vi "saveData.vi"(1 "display write dialog?":bool, 2 "append to file?":bool, 3 "Block Timing":T1) -> (0 "error out":errorcluster)   [LabVIEW 2013]
uses:
  Controls/blockTiming.ctl
  Globals/measurementGlobal.vi
panel:
  out "File Status":string="File not appended"
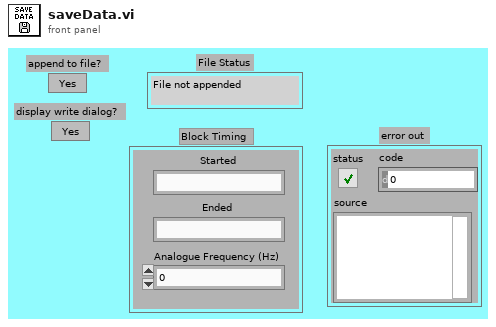
[diagram p1: front panel]
types:
  T1 = typedef "blockTiming.ctl" = cluster{"Started":string, "Ended":string, "Analogue Frequency (Hz)":dbl}
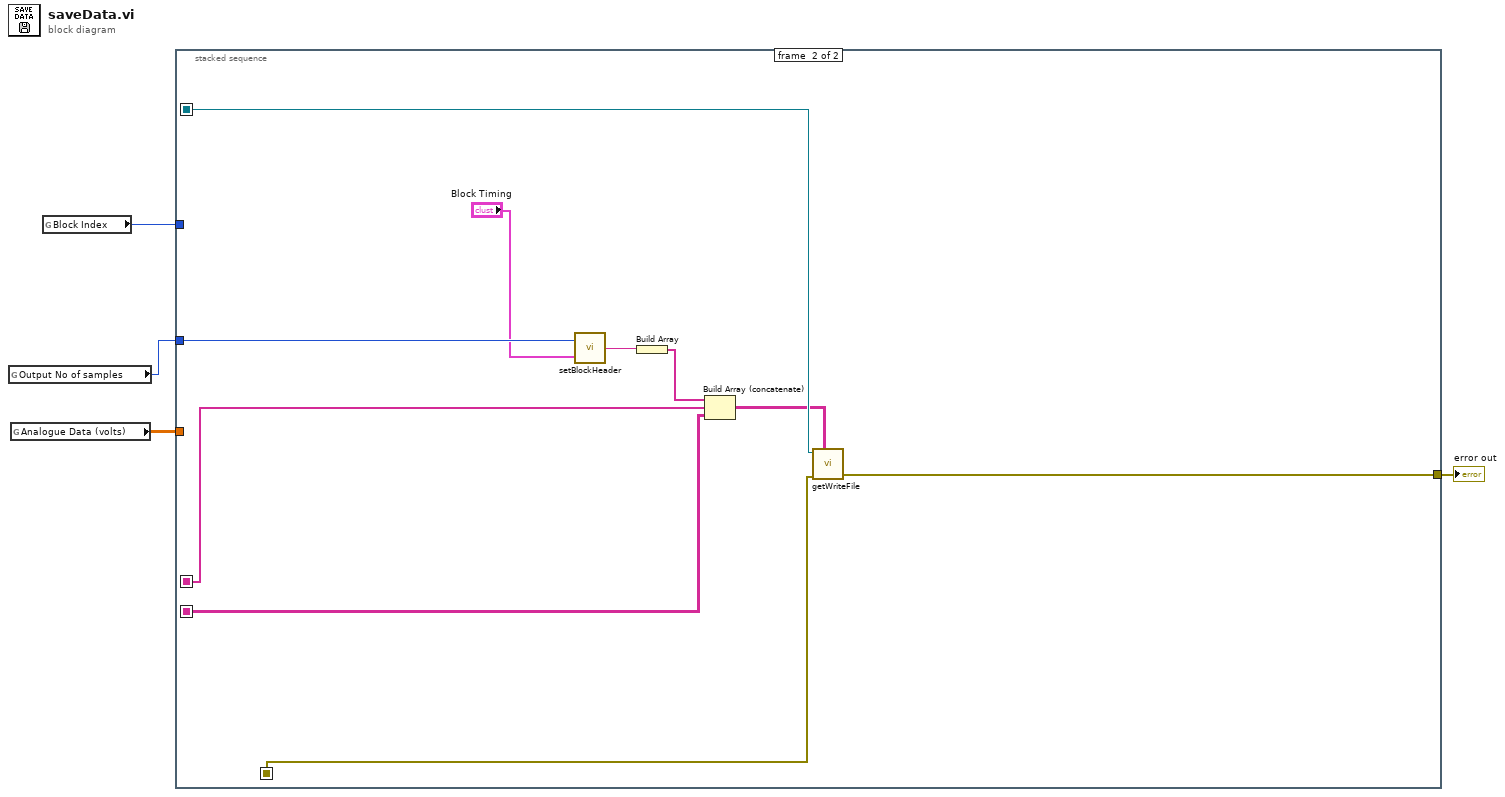
[diagram p0: block diagram]
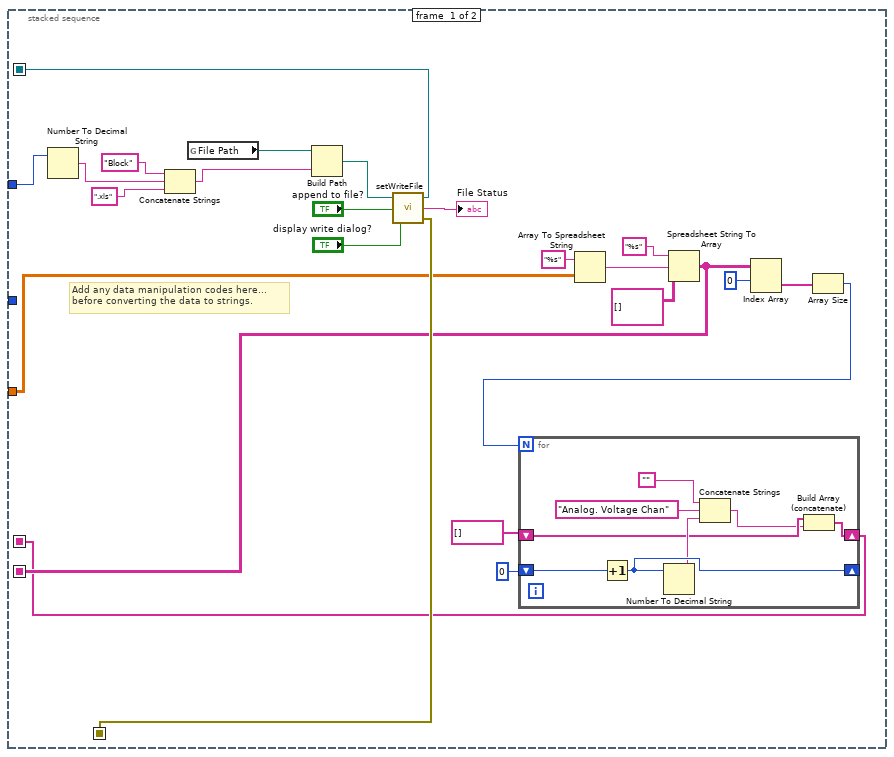
[diagram p2: hidden frame]
diagram:
  n1 = global read "measurementGlobal.vi" "Output No of samples"() -> (w3:i32)
  n2 = global read "measurementGlobal.vi" "Analogue Data (volts)"() -> (w4:dbl[][])
  n3 = global read "measurementGlobal.vi" "Block Index"() -> (w1:i32)
  n4 = stacked-sequence {
    seq-local: [w24 _] -> [_ w40]
    seq-local: [w23 _] -> [_ w39]
    seq-local: [w11 _] -> [_ w43]
    seq-local: [w10 _] -> [_ w44]
    tunnel: w4 -> [w19 _]
    tunnel: w3 -> [_ w46]
    tunnel: [_ w37] -> w2
    tunnel: w1 -> [w9 _]
    frame #0 {
      # "Add any data manipulation codes here... \nbefore converting the data to strings."
      n5 = Number To Decimal String(number=w9) -> (decimal integer string=w7:string)  [unwired: 1 in]
      n6 = Concatenate Strings("Block", w7, ".xls") -> (w5:string)
      n7 = global read "measurementGlobal.vi" "File Path"() -> (w28:path)
      n8 = Build Path(base path=w28, name or relative path=w5) -> (appended path=w27:path)
      n9 = call "setWriteFile.vi"("display write dialog?"="display write dialog?", "append to file?"="append to file?", "file path"=w27) -> ("error out"=w23:errorcluster, "Status"=→"File Status":string, "File Refnum"=w24:refnum<file>)
      n10 = Array To Spreadsheet String(array=w19, 3:"%s" ("format string")) -> (spreadsheet string=w15:string)  [unwired: 1 in]
      n11 = Spreadsheet String To Array(format string="%s", spreadsheet string=w15, array type (2D Dbl)=string[][] []) -> (array=w11:string[][])  [unwired: 1 in]
      n12 = Index Array(array=w11, index (row)=0) -> (element=w17:string[])  [unwired: 1 in]
      n13 = Array Size(array=w17) -> (size(s)=w16:i32)
      n14 = for {
        N: w16 -> [_]
        shift-right: [w35] -> _
        shift-left: 0 -> [w36]
        shift-right: [w29] -> w10
        shift-left: string[] [] -> [w32]
        n15 = Increment(x=w36) -> (x+1=w35:i32)
        n16 = Number To Decimal String(number=w35) -> (decimal integer string=w33:string)  [unwired: 1 in]
        n17 = Concatenate Strings("", "Analog. Voltage Chan" ("string"), w33) -> (w30:string)
        n18 = Build Array (concatenate)(w32, w30) -> (w29:string[])
      }
    }
    frame #1 {
      n19 = call "setBlockHeader.vi"("Block Timing"="Block Timing", "No of Analog. Samples"=w46) -> ("Output String"=w42:string)
      n20 = Build Array(w42) -> (w41:string[])
      n21 = Build Array (concatenate)(w41, w44, w43) -> (w38:string[][])
      n22 = call "getWriteFile.vi"("refnum in"=w40, "error in"=w39, "Data"=w38) -> ("error out"=w37:errorcluster)  [unwired: 2 in, 2 out]
    }
  }
  "error out" <- w2
